vi "BroadcastData.vi"(10 "Data":T1, 11 "通知器输入":refnum<notifier>) -> (3 "通知器输出":refnum<notifier>)   [LabVIEW 2018, in "DataDisplay.lvlib"]
uses:
  DataDisplay.lvlib
  TypeDefine/DD_DataStream.ctl
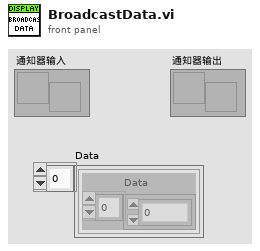
[diagram p1: front panel]
types:
  T1 = typedef "DataDisplay.lvlib/DD_DataStream.ctl" = cluster{"Data":dbl[]}[]
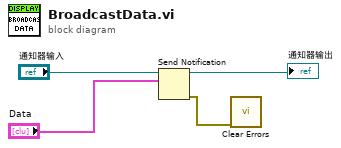
[diagram p0: block diagram]
diagram:
  n1 = Send Notification(notification="Data", notifier="通知器输入") -> (notifier out=→"通知器输出":refnum<notifier>, error out=w1:errorcluster)  [unwired: 1 in]
  n2 = call <vilib>:"Clear Errors.vi"("error in (no error)"=w1) -> ()  [unwired: 5 in, 2 out]
